vi "TCPClient.vi"() -> ()   [LabVIEW 2018]
panel:
  out "error out":errorcluster
  in  "Server Closed":string="The server VI closed the connection."
  in  "Stop":bool
  out "Waveform Graph":dbl[](graph)
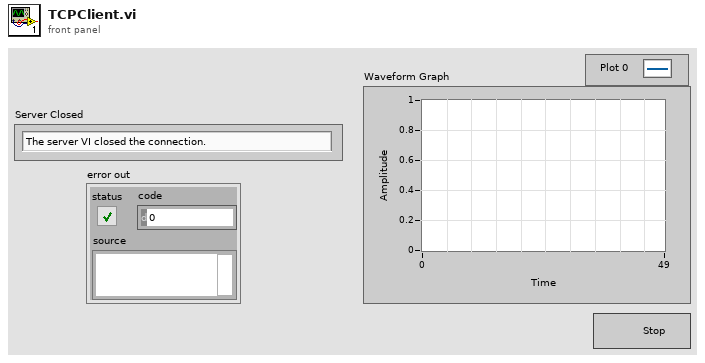
[diagram p1: front panel]
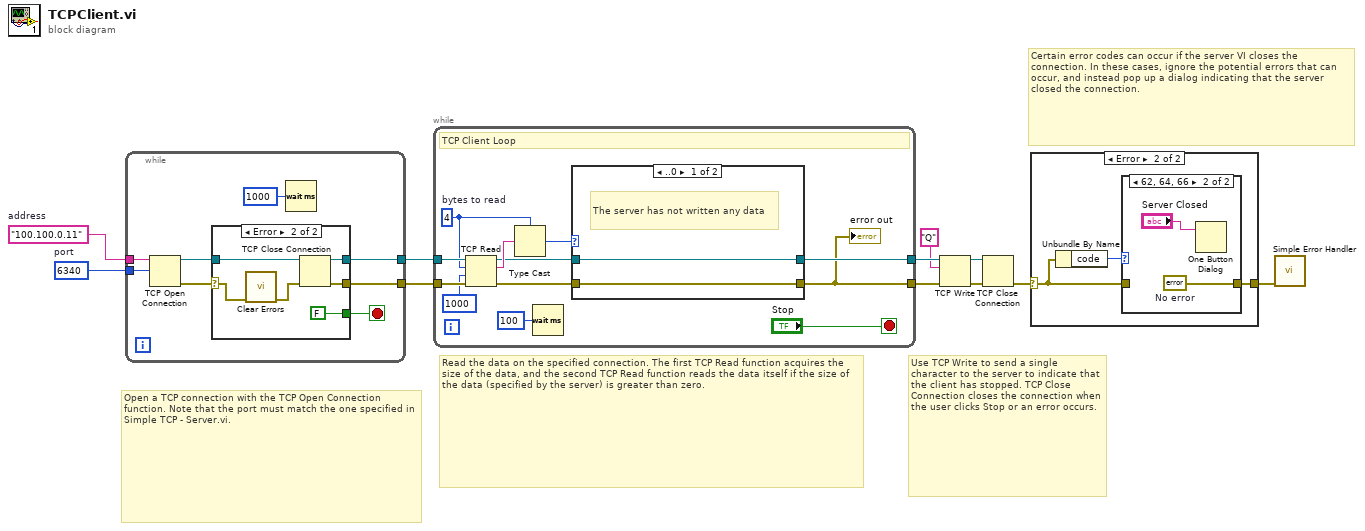
[diagram p0: block diagram]
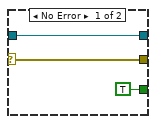
[diagram p2: hidden frame]
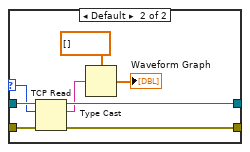
[diagram p5: hidden frame]
diagram:
  w4 = u16 6340  # port
  w3 = "100.100.0.11"  # address
  # "Certain error codes can occur if the server VI closes the connection. In these cases, ignore the potential errors that can occur, and instead pop up a dialog indicating that the server closed the connection."
  # "Use TCP Write to send a single character to the server to indicate that the client has stopped. TCP Close Connection closes the connection when the user clicks Stop or an error occurs."
  # "Read the data on the specified connection. The first TCP Read function acquires the size of the data, and the second TCP Read function reads the data itself if the size of the data (specified by the server) is greater than zero."
  # "Open a TCP connection with the TCP Open Connection function. Note that the port must match the one specified in Simple TCP - Server.vi."
  n1 = while {
    tunnel: [w16] -> w2
    tunnel: [w15] -> w1
    tunnel: w4 -> [w14]
    tunnel: w3 -> [w13]
    stop <- w17 stop-if-true
    n2 = TCP Open Connection(address=w13, remote port or service name=w14) -> (connection ID=w19:refnum<k5>, error out=w18:errorcluster)  [unwired: 3 in]
    n3 = case shown="Error" w18 {
      selector: w18 -> [w20 w27]
      tunnel: w19 -> [w21 w28]
      tunnel: [TRUE FALSE] -> w17
      tunnel: [w21 w24] -> w16
      tunnel: [w20 w23] -> w15
      frame No Error {
      }
      frame Error {
        n4 = call <vilib>:"Clear Errors.vi"("error in (no error)"=w27) -> ("error out"=w26:errorcluster)  [unwired: 5 in, 1 out]
        n5 = TCP Close Connection(connection ID=w28, error in (no error)=w26) -> (connection ID out=w24:refnum<k5>, error out=w23:errorcluster)  [unwired: 1 in]
      }
    }
    n6 = Wait (ms)(milliseconds to wait=u32 1000) -> ()  [unwired: 1 out]
  }
  n7 = while {
    tunnel: w1 -> [w36]
    tunnel: w2 -> [w37]
    tunnel: [w33] -> w10
    tunnel: [w32] -> w8
    stop <- "Stop" stop-if-true
    w35 = 4  # bytes to read
    # "TCP Client Loop"
    n8 = TCP Read(connection ID=w37, bytes to read=w35, error in (no error)=w36, 9:1000 ("timeout ms (25000)")) -> (connection ID out=w39:refnum<k5>, data out=w40:string, error out=w38:errorcluster)  [unwired: 1 in]
    n9 = Type Cast(type=w35, x=w40) -> (*(type *) &x=w31:i32)
    n10 = Wait (ms)(milliseconds to wait=u32 100) -> ()  [unwired: 1 out]
    n11 = case shown="..0" w31 {
      selector: w31 -> [_ w43]
      tunnel: w39 -> [w42 w50]
      tunnel: w38 -> [w41 w49]
      tunnel: [w42 w46] -> w33
      tunnel: [w41 w45] -> w32
      frame ..0 {
        # "The server has not written any data"
      }
      frame Default {
        n12 = TCP Read(connection ID=w50, bytes to read=w43, error in (no error)=w49) -> (connection ID out=w46:refnum<k5>, data out=w44:string, error out=w45:errorcluster)  [unwired: 2 in]
        n13 = Type Cast(type=dbl[] [] ("chart"), x=w44) -> (*(type *) &x=→"Waveform Graph":dbl[])
      }
    }
    "error out" <- w32
  }
  n14 = TCP Write(connection ID=w10, data in="Q", error in (no error)=w8) -> (connection ID out=w11:refnum<k5>, error out=w9:errorcluster)  [unwired: 2 out]
  n15 = TCP Close Connection(connection ID=w11, error in (no error)=w9) -> (error out=w6:errorcluster)  [unwired: 1 in, 1 out]
  n16 = case shown="Error" w6 {
    selector: w6 -> [w51 w53]
    tunnel: [w51 w52] -> w5
    frame No Error {
    }
    frame Error {
      n17 = Unbundle By Name(w53) -> ("code"=w54:i32)
      n18 = case shown="62, 64, 66" w54 {
        tunnel: w53 -> [w55 _]
        tunnel: [w55 w57] -> w52
        frame Default {
        }
        frame 62, 64, 66 {
          w57 = errorcluster {"status"=FALSE, "code"=0, "source"=""}  # No error
          n19 = One Button Dialog(message="Server Closed") -> ()  [unwired: 1 in, 1 out]
        }
      }
    }
  }
  n20 = call <vilib>:"Simple Error Handler.vi"("error in (no error)"=w5) -> ()  [unwired: 4 in, 5 out]
